vi "DDS_Clock.vi"() -> ()   [LabVIEW 2016] (continued)
"f1 [Hz] CH0"=318199999.99999994}, {"total time[ms]"=75.44999999999786, "f1 [Hz] CH0"=318199999.99999994}, {"total time[ms]"=75.49999999999785, "f1 [Hz] CH0"=318000000.0}, {"total time[ms]"=75.49999999999785, "f1 [Hz] CH0"=318000000.0}, {"total time[ms]"=75.54999999999785, "f1 [Hz] CH0"=317800000.0}, {"total time[ms]"=75.54999999999785, "f1 [Hz] CH0"=317800000.0}, {"total time[ms]"=75.59999999999785, "f1 [Hz] CH0"=317599999.99999994}, {"total time[ms]"=75.59999999999785, "f1 [Hz] CH0"=317599999.99999994}, {"total time[ms]"=75.64999999999785, "f1 [Hz] CH0"=317399999.99999994}, {"total time[ms]"=75.64999999999785, "f1 [Hz] CH0"=317399999.99999994}, {"total time[ms]"=75.69999999999784, "f1 [Hz] CH0"=317200000.0}, {"total time[ms]"=75.69999999999784, "f1 [Hz] CH0"=317200000.0}, {"total time[ms]"=75.74999999999784, "f1 [Hz] CH0"=317000000.0}, {"total time[ms]"=75.74999999999784, "f1 [Hz] CH0"=317000000.0}, {"total time[ms]"=75.79999999999784, "f1 [Hz] CH0"=316800000.0}, {"total time[ms]"=75.79999999999784, "f1 [Hz] CH0"=316800000.0}, {"total time[ms]"=75.84999999999783, "f1 [Hz] CH0"=316599999.99999994}, {"total time[ms]"=75.84999999999783, "f1 [Hz] CH0"=316599999.99999994}, {"total time[ms]"=75.89999999999783, "f1 [Hz] CH0"=316400000.0}, {"total time[ms]"=75.89999999999783, "f1 [Hz] CH0"=316400000.0}, {"total time[ms]"=75.94999999999783, "f1 [Hz] CH0"=316200000.0}, {"total time[ms]"=75.94999999999783, "f1 [Hz] CH0"=316200000.0}, {"total time[ms]"=75.99999999999783, "f1 [Hz] CH0"=316000000.0}, {"total time[ms]"=75.99999999999783, "f1 [Hz] CH0"=316000000.0}, {"total time[ms]"=76.04999999999782, "f1 [Hz] CH0"=315800000.0}, {"total time[ms]"=76.04999999999782, "f1 [Hz] CH0"=315800000.0}, {"total time[ms]"=76.09999999999782, "f1 [Hz] CH0"=315599999.99999994}, {"total time[ms]"=76.09999999999782, "f1 [Hz] CH0"=315599999.99999994}, {"total time[ms]"=76.14999999999782, "f1 [Hz] CH0"=315399999.99999994}, {"total time[ms]"=76.14999999999782, "f1 [Hz] CH0"=315399999.99999994}, {"total time[ms]"=76.19999999999781, "f1 [Hz] CH0"=315199999.99999994}, {"total time[ms]"=76.19999999999781, "f1 [Hz] CH0"=315199999.99999994}, {"total time[ms]"=76.24999999999781, "f1 [Hz] CH0"=315000000.0}, {"total time[ms]"=76.24999999999781, "f1 [Hz] CH0"=315000000.0}, {"total time[ms]"=76.29999999999781, "f1 [Hz] CH0"=314800000.0}, {"total time[ms]"=76.29999999999781, "f1 [Hz] CH0"=314800000.0}, {"total time[ms]"=76.3499999999978, "f1 [Hz] CH0"=314599999.99999994}, {"total time[ms]"=76.3499999999978, "f1 [Hz] CH0"=314599999.99999994}, {"total time[ms]"=76.3999999999978, "f1 [Hz] CH0"=314400000.0}, {"total time[ms]"=76.3999999999978, "f1 [Hz] CH0"=314400000.0}, {"total time[ms]"=76.4499999999978, "f1 [Hz] CH0"=314200000.0}, {"total time[ms]"=76.4499999999978, "f1 [Hz] CH0"=314200000.0}, {"total time[ms]"=76.4999999999978, "f1 [Hz] CH0"=314000000.0}, {"total time[ms]"=76.4999999999978, "f1 [Hz] CH0"=314000000.0}, {"total time[ms]"=76.5499999999978, "f1 [Hz] CH0"=313800000.0}, {"total time[ms]"=76.5499999999978, "f1 [Hz] CH0"=313800000.0}, {"total time[ms]"=76.59999999999779, "f1 [Hz] CH0"=313599999.99999994}, {"total time[ms]"=76.59999999999779, "f1 [Hz] CH0"=313599999.99999994}, {"total time[ms]"=76.64999999999779, "f1 [Hz] CH0"=313399999.99999994}, {"total time[ms]"=76.64999999999779, "f1 [Hz] CH0"=313399999.99999994}, {"total time[ms]"=76.69999999999779, "f1 [Hz] CH0"=313199999.99999994}, {"total time[ms]"=76.69999999999779, "f1 [Hz] CH0"=313199999.99999994}, {"total time[ms]"=76.74999999999778, "f1 [Hz] CH0"=313000000.0}, {"total time[ms]"=76.74999999999778, "f1 [Hz] CH0"=313000000.0}, {"total time[ms]"=76.79999999999778, "f1 [Hz] CH0"=312799999.99999994}, {"total time[ms]"=76.79999999999778, "f1 [Hz] CH0"=312799999.99999994}, {"total time[ms]"=76.84999999999778, "f1 [Hz] CH0"=312599999.99999994}, {"total time[ms]"=76.84999999999778, "f1 [Hz] CH0"=312599999.99999994}, {"total time[ms]"=76.89999999999777, "f1 [Hz] CH0"=312399999.99999994}, {"total time[ms]"=76.89999999999777, "f1 [Hz] CH0"=312399999.99999994}, {"total time[ms]"=76.94999999999777, "f1 [Hz] CH0"=312200000.0}, {"total time[ms]"=76.94999999999777, "f1 [Hz] CH0"=312200000.0}, {"total time[ms]"=76.99999999999777, "f1 [Hz] CH0"=312000000.0}, {"total time[ms]"=76.99999999999777, "f1 [Hz] CH0"=312000000.0}, {"total time[ms]"=77.04999999999777, "f1 [Hz] CH0"=311799999.99999994}, {"total time[ms]"=77.04999999999777, "f1 [Hz] CH0"=311799999.99999994}, {"total time[ms]"=77.09999999999776, "f1 [Hz] CH0"=311599999.99999994}, {"total time[ms]"=77.09999999999776, "f1 [Hz] CH0"=311599999.99999994}, {"total time[ms]"=77.14999999999776, "f1 [Hz] CH0"=311400000.0}, {"total time[ms]"=77.14999999999776, "f1 [Hz] CH0"=311400000.0}, {"total time[ms]"=77.19999999999776, "f1 [Hz] CH0"=311200000.0}, {"total time[ms]"=77.19999999999776, "f1 [Hz] CH0"=311200000.0}, {"total time[ms]"=77.24999999999775, "f1 [Hz] CH0"=311000000.0}, {"total time[ms]"=77.24999999999775, "f1 [Hz] CH0"=311000000.0}, {"total time[ms]"=77.29999999999775, "f1 [Hz] CH0"=310799999.99999994}, {"total time[ms]"=77.29999999999775, "f1 [Hz] CH0"=310799999.99999994}, {"total time[ms]"=77.34999999999775, "f1 [Hz] CH0"=310599999.99999994}, {"total time[ms]"=77.34999999999775, "f1 [Hz] CH0"=310599999.99999994}, {"total time[ms]"=77.39999999999775, "f1 [Hz] CH0"=310399999.99999994}, {"total time[ms]"=77.39999999999775, "f1 [Hz] CH0"=310399999.99999994}, {"total time[ms]"=77.44999999999774, "f1 [Hz] CH0"=310199999.99999994}, {"total time[ms]"=77.44999999999774, "f1 [Hz] CH0"=310199999.99999994}, {"total time[ms]"=77.49999999999774, "f1 [Hz] CH0"=310000000.0}, {"total time[ms]"=77.49999999999774, "f1 [Hz] CH0"=310000000.0}, {"total time[ms]"=77.54999999999774, "f1 [Hz] CH0"=309799999.99999994}, {"total time[ms]"=77.54999999999774, "f1 [Hz] CH0"=309799999.99999994}, {"total time[ms]"=77.59999999999773, "f1 [Hz] CH0"=309599999.99999994}, {"total time[ms]"=77.59999999999773, "f1 [Hz] CH0"=309599999.99999994}, {"total time[ms]"=77.64999999999773, "f1 [Hz] CH0"=309400000.0}, {"total time[ms]"=77.64999999999773, "f1 [Hz] CH0"=309400000.0}, {"total time[ms]"=77.69999999999773, "f1 [Hz] CH0"=309200000.0}, {"total time[ms]"=77.69999999999773, "f1 [Hz] CH0"=309200000.0}, {"total time[ms]"=77.74999999999773, "f1 [Hz] CH0"=309000000.0}, {"total time[ms]"=77.74999999999773, "f1 [Hz] CH0"=309000000.0}, {"total time[ms]"=77.79999999999772, "f1 [Hz] CH0"=308799999.99999994}, {"total time[ms]"=77.79999999999772, "f1 [Hz] CH0"=308799999.99999994}, {"total time[ms]"=77.84999999999772, "f1 [Hz] CH0"=308599999.99999994}, {"total time[ms]"=77.84999999999772, "f1 [Hz] CH0"=308599999.99999994}, {"total time[ms]"=77.89999999999772, "f1 [Hz] CH0"=308399999.99999994}, {"total time[ms]"=77.89999999999772, "f1 [Hz] CH0"=308399999.99999994}, {"total time[ms]"=77.94999999999771, "f1 [Hz] CH0"=308199999.99999994}, {"total time[ms]"=77.94999999999771, "f1 [Hz] CH0"=308199999.99999994}, {"total time[ms]"=77.99999999999771, "f1 [Hz] CH0"=308000000.0}, {"total time[ms]"=77.99999999999771, "f1 [Hz] CH0"=308000000.0}, {"total time[ms]"=78.04999999999771, "f1 [Hz] CH0"=307799999.99999994}, {"total time[ms]"=78.04999999999771, "f1 [Hz] CH0"=307799999.99999994}, {"total time[ms]"=78.0999999999977, "f1 [Hz] CH0"=307599999.99999994}, {"total time[ms]"=78.0999999999977, "f1 [Hz] CH0"=307599999.99999994}, {"total time[ms]"=78.1499999999977, "f1 [Hz] CH0"=307399999.99999994}, {"total time[ms]"=78.1499999999977, "f1 [Hz] CH0"=307399999.99999994}, {"total time[ms]"=78.1999999999977, "f1 [Hz] CH0"=307200000.0}, {"total time[ms]"=78.1999999999977, "f1 [Hz] CH0"=307200000.0}, {"total time[ms]"=78.2499999999977, "f1 [Hz] CH0"=307000000.0}, {"total time[ms]"=78.2499999999977, "f1 [Hz] CH0"=307000000.0}, {"total time[ms]"=78.2999999999977, "f1 [Hz] CH0"=306799999.99999994}, {"total time[ms]"=78.2999999999977, "f1 [Hz] CH0"=306799999.99999994}, {"total time[ms]"=78.34999999999769, "f1 [Hz] CH0"=306599999.99999994}, {"total time[ms]"=78.34999999999769, "f1 [Hz] CH0"=306599999.99999994}, {"total time[ms]"=78.39999999999769, "f1 [Hz] CH0"=306400000.0}, {"total time[ms]"=78.39999999999769, "f1 [Hz] CH0"=306400000.0}, {"total time[ms]"=78.44999999999769, "f1 [Hz] CH0"=306200000.0}, {"total time[ms]"=78.44999999999769, "f1 [Hz] CH0"=306200000.0}, {"total time[ms]"=78.49999999999768, "f1 [Hz] CH0"=306000000.0}, {"total time[ms]"=78.49999999999768, "f1 [Hz] CH0"=306000000.0}, {"total time[ms]"=78.54999999999768, "f1 [Hz] CH0"=305799999.99999994}, {"total time[ms]"=78.54999999999768, "f1 [Hz] CH0"=305799999.99999994}, {"total time[ms]"=78.59999999999768, "f1 [Hz] CH0"=305599999.99999994}, {"total time[ms]"=78.59999999999768, "f1 [Hz] CH0"=305599999.99999994}, {"total time[ms]"=78.64999999999768, "f1 [Hz] CH0"=305399999.99999994}, {"total time[ms]"=78.64999999999768, "f1 [Hz] CH0"=305399999.99999994}, {"total time[ms]"=78.69999999999767, "f1 [Hz] CH0"=305199999.99999994}, {"total time[ms]"=78.69999999999767, "f1 [Hz] CH0"=305199999.99999994}, {"total time[ms]"=78.74999999999767, "f1 [Hz] CH0"=305000000.0}, {"total time[ms]"=78.74999999999767, "f1 [Hz] CH0"=305000000.0}, {"total time[ms]"=78.79999999999767, "f1 [Hz] CH0"=304799999.99999994}, {"total time[ms]"=78.79999999999767, "f1 [Hz] CH0"=304799999.99999994}, {"total time[ms]"=78.84999999999766, "f1 [Hz] CH0"=304599999.99999994}, {"total time[ms]"=78.84999999999766, "f1 [Hz] CH0"=304599999.99999994}, {"total time[ms]"=78.89999999999766, "f1 [Hz] CH0"=304400000.0}, {"total time[ms]"=78.89999999999766, "f1 [Hz] CH0"=304400000.0}, {"total time[ms]"=78.94999999999766, "f1 [Hz] CH0"=304200000.0}, {"total time[ms]"=78.94999999999766, "f1 [Hz] CH0"=304200000.0}, {"total time[ms]"=78.99999999999766, "f1 [Hz] CH0"=304000000.0}, {"total time[ms]"=78.99999999999766, "f1 [Hz] CH0"=304000000.0}, {"total time[ms]"=79.04999999999765, "f1 [Hz] CH0"=303799999.99999994}, {"total time[ms]"=79.04999999999765, "f1 [Hz] CH0"=303799999.99999994}, {"total time[ms]"=79.09999999999765, "f1 [Hz] CH0"=303599999.99999994}, {"total time[ms]"=79.09999999999765, "f1 [Hz] CH0"=303599999.99999994}, {"total time[ms]"=79.14999999999765, "f1 [Hz] CH0"=303399999.99999994}, {"total time[ms]"=79.14999999999765, "f1 [Hz] CH0"=303399999.99999994}, {"total time[ms]"=79.19999999999764, "f1 [Hz] CH0"=303199999.99999994}, {"total time[ms]"=79.19999999999764, "f1 [Hz] CH0"=303199999.99999994}, {"total time[ms]"=79.24999999999764, "f1 [Hz] CH0"=303000000.0}, {"total time[ms]"=79.24999999999764, "f1 [Hz] CH0"=303000000.0}, {"total time[ms]"=79.29999999999764, "f1 [Hz] CH0"=302799999.99999994}, {"total time[ms]"=79.29999999999764, "f1 [Hz] CH0"=302799999.99999994}, {"total time[ms]"=79.34999999999764, "f1 [Hz] CH0"=302599999.99999994}, {"total time[ms]"=79.34999999999764, "f1 [Hz] CH0"=302599999.99999994}, {"total time[ms]"=79.39999999999763, "f1 [Hz] CH0"=302399999.99999994}, {"total time[ms]"=79.39999999999763, "f1 [Hz] CH0"=302399999.99999994}, {"total time[ms]"=79.44999999999763, "f1 [Hz] CH0"=302200000.0}, {"total time[ms]"=79.44999999999763, "f1 [Hz] CH0"=302200000.0}, {"total time[ms]"=79.49999999999763, "f1 [Hz] CH0"=302000000.0}, {"total time[ms]"=79.49999999999763, "f1 [Hz] CH0"=302000000.0}, {"total time[ms]"=79.54999999999762, "f1 [Hz] CH0"=301799999.99999994}, {"total time[ms]"=79.54999999999762, "f1 [Hz] CH0"=301799999.99999994}, {"total time[ms]"=79.59999999999762, "f1 [Hz] CH0"=301599999.99999994}, {"total time[ms]"=79.59999999999762, "f1 [Hz] CH0"=301599999.99999994}, {"total time[ms]"=79.64999999999762, "f1 [Hz] CH0"=301400000.0}, {"total time[ms]"=79.64999999999762, "f1 [Hz] CH0"=301400000.0}, {"total time[ms]"=79.69999999999762, "f1 [Hz] CH0"=301200000.0}, {"total time[ms]"=79.69999999999762, "f1 [Hz] CH0"=301200000.0}, {"total time[ms]"=79.74999999999761, "f1 [Hz] CH0"=301000000.0}, {"total time[ms]"=79.74999999999761, "f1 [Hz] CH0"=301000000.0}, {"total time[ms]"=79.79999999999761, "f1 [Hz] CH0"=300799999.99999994}, {"total time[ms]"=79.79999999999761, "f1 [Hz] CH0"=300799999.99999994}, {"total time[ms]"=79.8499999999976, "f1 [Hz] CH0"=300599999.99999994}, {"total time[ms]"=79.8499999999976, "f1 [Hz] CH0"=300599999.99999994}, {"total time[ms]"=79.8999999999976, "f1 [Hz] CH0"=300399999.99999994}, {"total time[ms]"=79.8999999999976, "f1 [Hz] CH0"=300399999.99999994}, {"total time[ms]"=79.9499999999976, "f1 [Hz] CH0"=300199999.99999994}, {"total time[ms]"=79.9499999999976, "f1 [Hz] CH0"=300199999.99999994}, {"total time[ms]"=79.9999999999976, "f1 [Hz] CH0"=300000000.0}, {"total time[ms]"=79.9999999999976, "f1 [Hz] CH0"=300000000.0}, {"total time[ms]"=80.0499999999976, "f1 [Hz] CH0"=300200000.00000006}, {"total time[ms]"=80.0499999999976, "f1 [Hz] CH0"=300200000.00000006}, {"total time[ms]"=80.09999999999759, "f1 [Hz] CH0"=300400000.00000006}, {"total time[ms]"=80.09999999999759, "f1 [Hz] CH0"=300400000.00000006}, {"total time[ms]"=80.14999999999759, "f1 [Hz] CH0"=300600000.0}, {"total time[ms]"=80.14999999999759, "f1 [Hz] CH0"=300600000.0}, {"total time[ms]"=80.19999999999759, "f1 [Hz] CH0"=300800000.00000006}, {"total time[ms]"=80.19999999999759, "f1 [Hz] CH0"=300800000.00000006}, {"total time[ms]"=80.24999999999758, "f1 [Hz] CH0"=301000000.0}, {"total time[ms]"=80.24999999999758, "f1 [Hz] CH0"=301000000.0}, {"total time[ms]"=80.29999999999758, "f1 [Hz] CH0"=301200000.00000006}, {"total time[ms]"=80.29999999999758, "f1 [Hz] CH0"=301200000.00000006}, {"total time[ms]"=80.34999999999758, "f1 [Hz] CH0"=301400000.00000006}, {"total time[ms]"=80.34999999999758, "f1 [Hz] CH0"=301400000.00000006}, {"total time[ms]"=80.39999999999758, "f1 [Hz] CH0"=301600000.00000006}, {"total time[ms]"=80.39999999999758, "f1 [Hz] CH0"=301600000.00000006}, {"total time[ms]"=80.44999999999757, "f1 [Hz] CH0"=301800000.0}, {"total time[ms]"=80.44999999999757, "f1 [Hz] CH0"=301800000.0}, {"total time[ms]"=80.49999999999757, "f1 [Hz] CH0"=302000000.0}, {"total time[ms]"=80.49999999999757, "f1 [Hz] CH0"=302000000.0}, {"total time[ms]"=80.54999999999757, "f1 [Hz] CH0"=302200000.00000006}, {"total time[ms]"=80.54999999999757, "f1 [Hz] CH0"=302200000.00000006}, {"total time[ms]"=80.59999999999756, "f1 [Hz] CH0"=302400000.0}, {"total time[ms]"=80.59999999999756, "f1 [Hz] CH0"=302400000.0}, {"total time[ms]"=80.64999999999756, "f1 [Hz] CH0"=302600000.00000006}, {"total time[ms]"=80.64999999999756, "f1 [Hz] CH0"=302600000.00000006}, {"total time[ms]"=80.69999999999756, "f1 [Hz] CH0"=302800000.0}, {"total time[ms]"=80.69999999999756, "f1 [Hz] CH0"=302800000.0}, {"total time[ms]"=80.74999999999756, "f1 [Hz] CH0"=303000000.00000006}, {"total time[ms]"=80.74999999999756, "f1 [Hz] CH0"=303000000.00000006}, {"total time[ms]"=80.79999999999755, "f1 [Hz] CH0"=303200000.00000006}, {"total time[ms]"=80.79999999999755, "f1 [Hz] CH0"=303200000.00000006}, {"total time[ms]"=80.84999999999755, "f1 [Hz] CH0"=303400000.00000006}, {"total time[ms]"=80.84999999999755, "f1 [Hz] CH0"=303400000.00000006}, {"total time[ms]"=80.89999999999755, "f1 [Hz] CH0"=303600000.00000006}, {"total time[ms]"=80.89999999999755, "f1 [Hz] CH0"=303600000.00000006}, {"total time[ms]"=80.94999999999754, "f1 [Hz] CH0"=303800000.0}, {"total time[ms]"=80.94999999999754, "f1 [Hz] CH0"=303800000.0}, {"total time[ms]"=80.99999999999754, "f1 [Hz] CH0"=304000000.0}, {"total time[ms]"=80.99999999999754, "f1 [Hz] CH0"=304000000.0}, {"total time[ms]"=81.04999999999754, "f1 [Hz] CH0"=304200000.00000006}, {"total time[ms]"=81.04999999999754, "f1 [Hz] CH0"=304200000.00000006}, {"total time[ms]"=81.09999999999754, "f1 [Hz] CH0"=304400000.00000006}, {"total time[ms]"=81.09999999999754, "f1 [Hz] CH0"=304400000.00000006}, {"total time[ms]"=81.14999999999753, "f1 [Hz] CH0"=304600000.0}, {"total time[ms]"=81.14999999999753, "f1 [Hz] CH0"=304600000.0}, {"total time[ms]"=81.19999999999753, "f1 [Hz] CH0"=304800000.00000006}, {"total time[ms]"=81.19999999999753, "f1 [Hz] CH0"=304800000.00000006}, {"total time[ms]"=81.24999999999753, "f1 [Hz] CH0"=305000000.0}, {"total time[ms]"=81.24999999999753, "f1 [Hz] CH0"=305000000.0}, {"total time[ms]"=81.29999999999752, "f1 [Hz] CH0"=305200000.00000006}, {"total time[ms]"=81.29999999999752, "f1 [Hz] CH0"=305200000.00000006}, {"total time[ms]"=81.34999999999752, "f1 [Hz] CH0"=305400000.00000006}, {"total time[ms]"=81.34999999999752, "f1 [Hz] CH0"=305400000.00000006}, {"total time[ms]"=81.39999999999752, "f1 [Hz] CH0"=305600000.0}, {"total time[ms]"=81.39999999999752, "f1 [Hz] CH0"=305600000.0}, {"total time[ms]"=81.44999999999752, "f1 [Hz] CH0"=305800000.00000006}, {"total time[ms]"=81.44999999999752, "f1 [Hz] CH0"=305800000.00000006}, {"total time[ms]"=81.49999999999751, "f1 [Hz] CH0"=306000000.0}, {"total time[ms]"=81.49999999999751, "f1 [Hz] CH0"=306000000.0}, {"total time[ms]"=81.54999999999751, "f1 [Hz] CH0"=306200000.00000006}, {"total time[ms]"=81.54999999999751, "f1 [Hz] CH0"=306200000.00000006}, {"total time[ms]"=81.59999999999751, "f1 [Hz] CH0"=306400000.00000006}, {"total time[ms]"=81.59999999999751, "f1 [Hz] CH0"=306400000.00000006}, {"total time[ms]"=81.6499999999975, "f1 [Hz] CH0"=306600000.00000006}, {"total time[ms]"=81.6499999999975, "f1 [Hz] CH0"=306600000.00000006}, {"total time[ms]"=81.6999999999975, "f1 [Hz] CH0"=306800000.0}, {"total time[ms]"=81.6999999999975, "f1 [Hz] CH0"=306800000.0}, {"total time[ms]"=81.7499999999975, "f1 [Hz] CH0"=307000000.0}, {"total time[ms]"=81.7499999999975, "f1 [Hz] CH0"=307000000.0}, {"total time[ms]"=81.7999999999975, "f1 [Hz] CH0"=307200000.00000006}, {"total time[ms]"=81.7999999999975, "f1 [Hz] CH0"=307200000.00000006}, {"total time[ms]"=81.8499999999975, "f1 [Hz] CH0"=307400000.0}, {"total time[ms]"=81.8499999999975, "f1 [Hz] CH0"=307400000.0}, {"total time[ms]"=81.89999999999749, "f1 [Hz] CH0"=307600000.00000006}, {"total time[ms]"=81.89999999999749, "f1 [Hz] CH0"=307600000.00000006}, {"total time[ms]"=81.94999999999749, "f1 [Hz] CH0"=307800000.0}, {"total time[ms]"=81.94999999999749, "f1 [Hz] CH0"=307800000.0}, {"total time[ms]"=81.99999999999748, "f1 [Hz] CH0"=308000000.00000006}, {"total time[ms]"=81.99999999999748, "f1 [Hz] CH0"=308000000.00000006}, {"total time[ms]"=82.04999999999748, "f1 [Hz] CH0"=308200000.00000006}, {"total time[ms]"=82.04999999999748, "f1 [Hz] CH0"=308200000.00000006}, {"total time[ms]"=82.09999999999748, "f1 [Hz] CH0"=308400000.00000006}, {"total time[ms]"=82.09999999999748, "f1 [Hz] CH0"=308400000.00000006}, {"total time[ms]"=82.14999999999748, "f1 [Hz] CH0"=308600000.00000006}, {"total time[ms]"=82.14999999999748, "f1 [Hz] CH0"=308600000.00000006}, {"total time[ms]"=82.19999999999747, "f1 [Hz] CH0"=308800000.0}, {"total time[ms]"=82.19999999999747, "f1 [Hz] CH0"=308800000.0}, {"total time[ms]"=82.24999999999747, "f1 [Hz] CH0"=309000000.0}, {"total time[ms]"=82.24999999999747, "f1 [Hz] CH0"=309000000.0}, {"total time[ms]"=82.29999999999747, "f1 [Hz] CH0"=309200000.00000006}, {"total time[ms]"=82.29999999999747, "f1 [Hz] CH0"=309200000.00000006}, {"total time[ms]"=82.34999999999746, "f1 [Hz] CH0"=309400000.00000006}, {"total time[ms]"=82.34999999999746, "f1 [Hz] CH0"=309400000.00000006}, {"total time[ms]"=82.39999999999746, "f1 [Hz] CH0"=309600000.0}, {"total time[ms]"=82.39999999999746, "f1 [Hz] CH0"=309600000.0}, {"total time[ms]"=82.44999999999746, "f1 [Hz] CH0"=309800000.00000006}, {"total time[ms]"=82.44999999999746, "f1 [Hz] CH0"=309800000.00000006}, {"total time[ms]"=82.49999999999746, "f1 [Hz] CH0"=310000000.0}, {"total time[ms]"=82.49999999999746, "f1 [Hz] CH0"=310000000.0}, {"total time[ms]"=82.54999999999745, "f1 [Hz] CH0"=310200000.00000006}, {"total time[ms]"=82.54999999999745, "f1 [Hz] CH0"=310200000.00000006}, {"total time[ms]"=82.59999999999745, "f1 [Hz] CH0"=310400000.00000006}, {"total time[ms]"=82.59999999999745, "f1 [Hz] CH0"=310400000.00000006}, {"total time[ms]"=82.64999999999745, "f1 [Hz] CH0"=310600000.0}, {"total time[ms]"=82.64999999999745, "f1 [Hz] CH0"=310600000.0}, {"total time[ms]"=82.69999999999744, "f1 [Hz] CH0"=310800000.00000006}, 
